vi "Delete Filter.vi"(0 "Display State In":T1={"logTable"=refnum, "max items"=500, "displaydata"=[], "data"=[], "Auto Scroll"=TRUE, "current item"=500, "col headers"=[], "Add to Top"=TRUE, "Auto resize"=TRUE, "col size"=[], "filters"=[], "color cells"=[]}, 5 "column":string, 9 "Container State":T3, 11 "error in (no error)":errorcluster) -> (4 "Display State Out":T1={"logTable"=refnum, "max items"=500, "displaydata"=[], "data"=[], "Auto Scroll"=TRUE, "current item"=500, "col headers"=[], "Add to Top"=TRUE, "Auto resize"=TRUE, "col size"=[], "filters"=[], "color cells"=[]}, 15 "error out":errorcluster)   [LabVIEW 2013, in "UI-DisplayTable(dev).xctl"]
uses:
  UI-DisplayTable(dev).xctl
  <vilib>/_xctls/Container State.ctl
  State.ctl
  Support/DEF-Filter.ctl
  <vilib>/_xctls/XControlSupport.lvlib
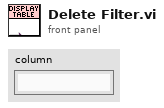
[diagram p1: front panel]
types:
  T1 = typedef "UI-DisplayTable(dev).xctl/State.ctl" = cluster{"logTable":refnum<vi>, "max items":i32, "displaydata":string[][], "data":string[][], "Auto Scroll":bool, "current item":i32, "col headers":string[], "Add to Top":bool, "Auto resize":bool, "col size":i32[], "filters":T2[], "color cells":cluster{"color cell":cluster{"Column":string, "Value":string, "Highlight Column":string}, "Color Box":u32}[]}
  T2 = typedef "UI-DisplayTable(dev).xctl/DEF-Filter.ctl" = cluster{"column":string, "value":string[]}
  T3 = typedef "XControlSupport.lvlib/Container State.ctl" = cluster{"Indicator?":bool, "Run Mode?":bool, " Refnum":refnum<vi>}
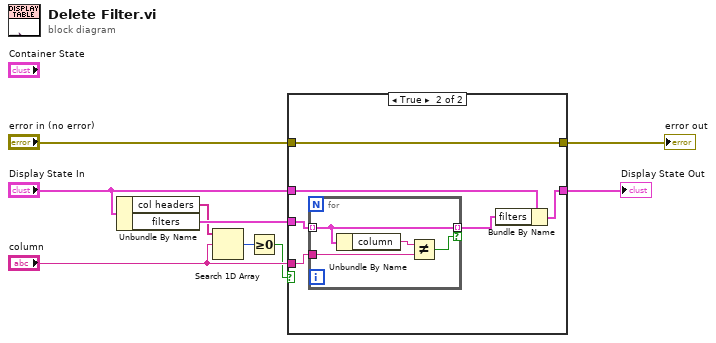
[diagram p0: block diagram]
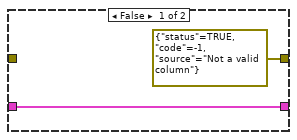
[diagram p2: hidden frame]
diagram:
  n1 = Unbundle By Name("Display State In") -> ("col headers"=w6:string[], "filters"=w9:T2[])
  n2 = Search 1D Array(1D array=w6, element="column") -> (index of element=w4:i32)  [unwired: 1 in]
  n3 = Greater Or Equal To 0?(x=w4) -> (x >= 0?=w3:bool)
  n4 = case shown="True" w3 {
    tunnel: w9 -> [_ w17]
    tunnel: "column" -> [_ w16]
    tunnel: "Display State In" -> [w11 w15]
    tunnel: [w11 w14] -> w7
    tunnel: "error in (no error)" -> [_ w12]
    tunnel: [errorcluster {"status"=TRUE, "code"=-1, "source"="Not a valid column"} ("error in (no error)") w12] -> w1
    frame False {
    }
    frame True {
      n5 = for {
        tunnel: w17 -> [w19] mode=indexing
        tunnel: w16 -> [w20]
        tunnel: [w19] -> w13 mode=indexing if=w18
        n6 = Unbundle By Name(w19) -> ("column"=w21:string)
        n7 = Not Equal?(x=w21, y=w20) -> (x != y?=w18:bool)
      }
      n8 = Bundle By Name(cluster=w15, "filters"=w13) -> (w14:T1)
    }
  }
  "Display State Out" <- w7
  "error out" <- w1
